vi "TEST - BUG ID 1501747.vi"(8 "error in (no error)":errorcluster) -> (0 "error out":errorcluster, 2 "Passed?":bool)   [LabVIEW 2020, in "test_openg_variant_config_file.lvlib"]
uses:
  <vilib>/addons/_JKI Toolkits/Caraya/classes/Assert/Assert True.vi
  test_openg_variant_config_file.lvlib
  <userlib>/_OpenG.lib/file/file.llb/openg_file.lvlib
  source/library/openg_variant_configuration_file.lvlib
  <vilib>/Utility/config.llb/NI_LVConfig.lvlib
  <vilib>/addons/_JKI Toolkits/Caraya/classes/Test/Test.lvclass
  <vilib>/addons/_JKI Toolkits/Caraya/classes/Assert/Assert.lvclass
panel:
  # "https://sourceforge.net/tracker/?func=detail&aid=1501747&group_id=52435&atid=466832"
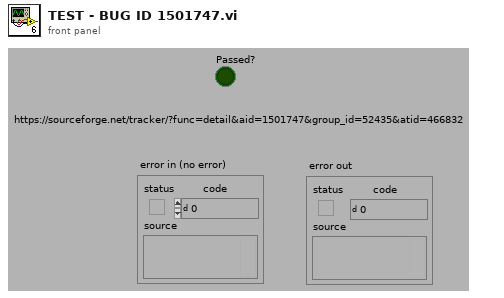
[diagram p1: front panel]
types:
  T1 = typedef "NI_LVConfig.lvlib/Config Data RefNum.ctl" = refnum<k1>
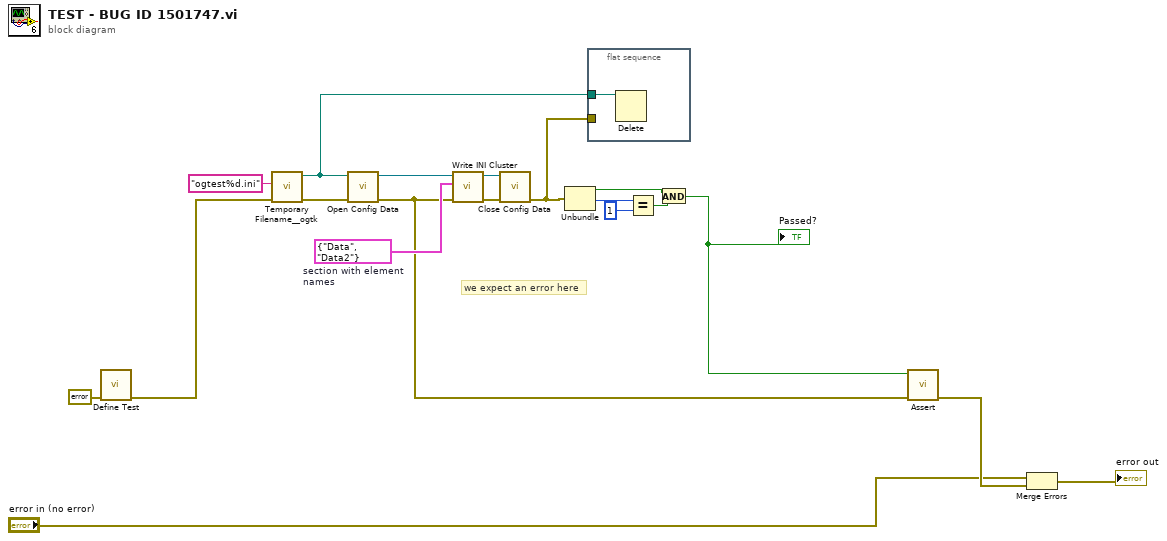
[diagram p0: block diagram]
diagram:
  w14 = cluster{string, string} {"Data", "Data2"}  # section with element names
  # "we expect an error here"
  n1 = call <vilib>:"Define Test.vi"("error in (no error)"=errorcluster {"status"=FALSE, "code"=0, "source"=""}) -> ("error out"=w5:errorcluster)  [unwired: 9 in, 1 out]
  n2 = call <userlib>:"Temporary Filename__ogtk.vi"("error in (no error)"=w5, "pattern (lvtemp%d.tmp)"="ogtest%d.ini") -> ("error out"=w15:errorcluster, "file in tmp dir"=w9:path)  [unwired: 4 in]
  n3 = call <vilib>:"Open Config Data.vi"("error in (no error)"=w15, "configuration file path"=w9) -> ("error out"=w3:errorcluster, "refnum"=w18:T1)  [unwired: 7 in, 1 out]
  n4 = call "Write INI Cluster.vi"("error in (no error)"=w3, "INI Fomatted Cluster"=w14, "refnum"=w18) -> ("error out"=w16:errorcluster, "dup refnum"=w17:T1)  [unwired: 7 in]
  n5 = call <vilib>:"Close Config Data.vi"("error in (no error)"=w16, "refnum"=w17) -> ("error out"=w8:errorcluster)  [unwired: 8 in, 1 out]
  n6 = Unbundle(w8) -> ("status"=w12:bool, "code"=w10:i32)  [unwired: 1 out]
  n7 = flat-sequence {
    tunnel: w9 -> [w20]
    tunnel: w8 -> [_]
    frame #0 {
      n8 = Delete(path (use dialog)=w20) -> ()  [unwired: 4 in, 3 out]
    }
  }
  n9 = Equal?(x=w10, y=1) -> (x = y?=w13:bool)
  n10 = And(x=w12, y=w13) -> (x .and. y?=w4:bool)
  "Passed?" <- w4
  n11 = call-poly <vilib>:"Assert.vi"("error in (no error)"=w3, "True?"=w4) -> ("error out"=w6:errorcluster)  [unwired: 8 in, 1 out]
  n12 = Merge Errors("error in (no error)", w6) -> (→"error out":errorcluster)
